vi "KeithsPhidgetAntennaOrientationFinal.vi"() -> ()   [LabVIEW 2016]
panel:
  out "Reference Elevation":sgl
  out "Reference Azimuth":dbl format="%#_13g"
  in  "Accept":bool
  in  "Don't Accept":bool
  out "Azimuth":dbl format="%#_13g"
  out "Measurements":dbl[][](array[numeric])
  in  "Antenna Power 2":dbl
  in  "Measure 2":bool
  in  "END":bool
  out "Event? 2":bool
  out "Elevation":dbl format="%#_13g"
  out "error out 2":errorcluster
  out "Attached? 2":bool
  out "Serial Number 2":i32
  in  "Antenna Power":dbl
  in  "Home":bool
  in  "Measure":bool
  out "error out":errorcluster
  out "Event?":bool
  out "Attached?":bool
  out "Serial Number":i32
  # "Reference Azimuth and Elevation"
  # "Azimuth, Elevation and Power"
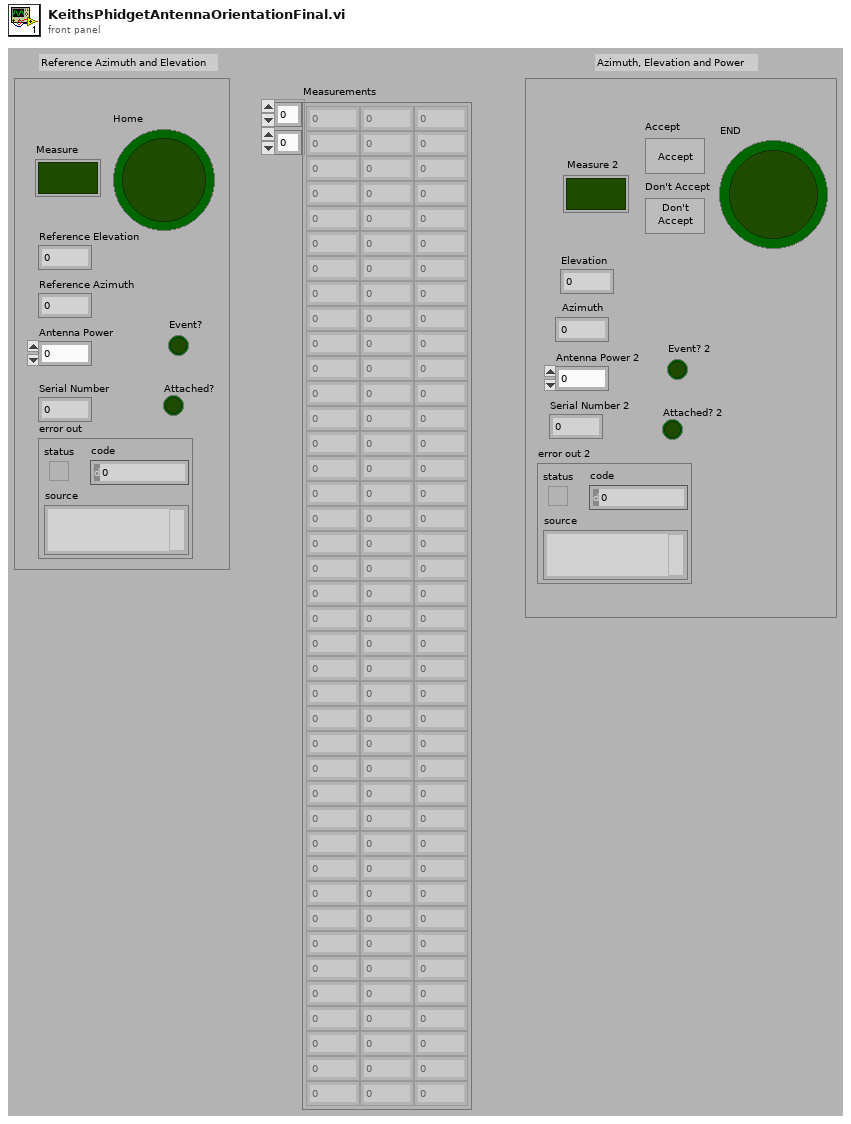
[diagram p1: front panel]
types:
  T1 = cluster{"acc0":dbl, "acc1":dbl, "acc3":dbl, "ang0":dbl, "ang1":dbl, "ang2":dbl, "mag0":dbl, "mag1":dbl, "mag2":dbl, "sec":i32, "micsec":i32}
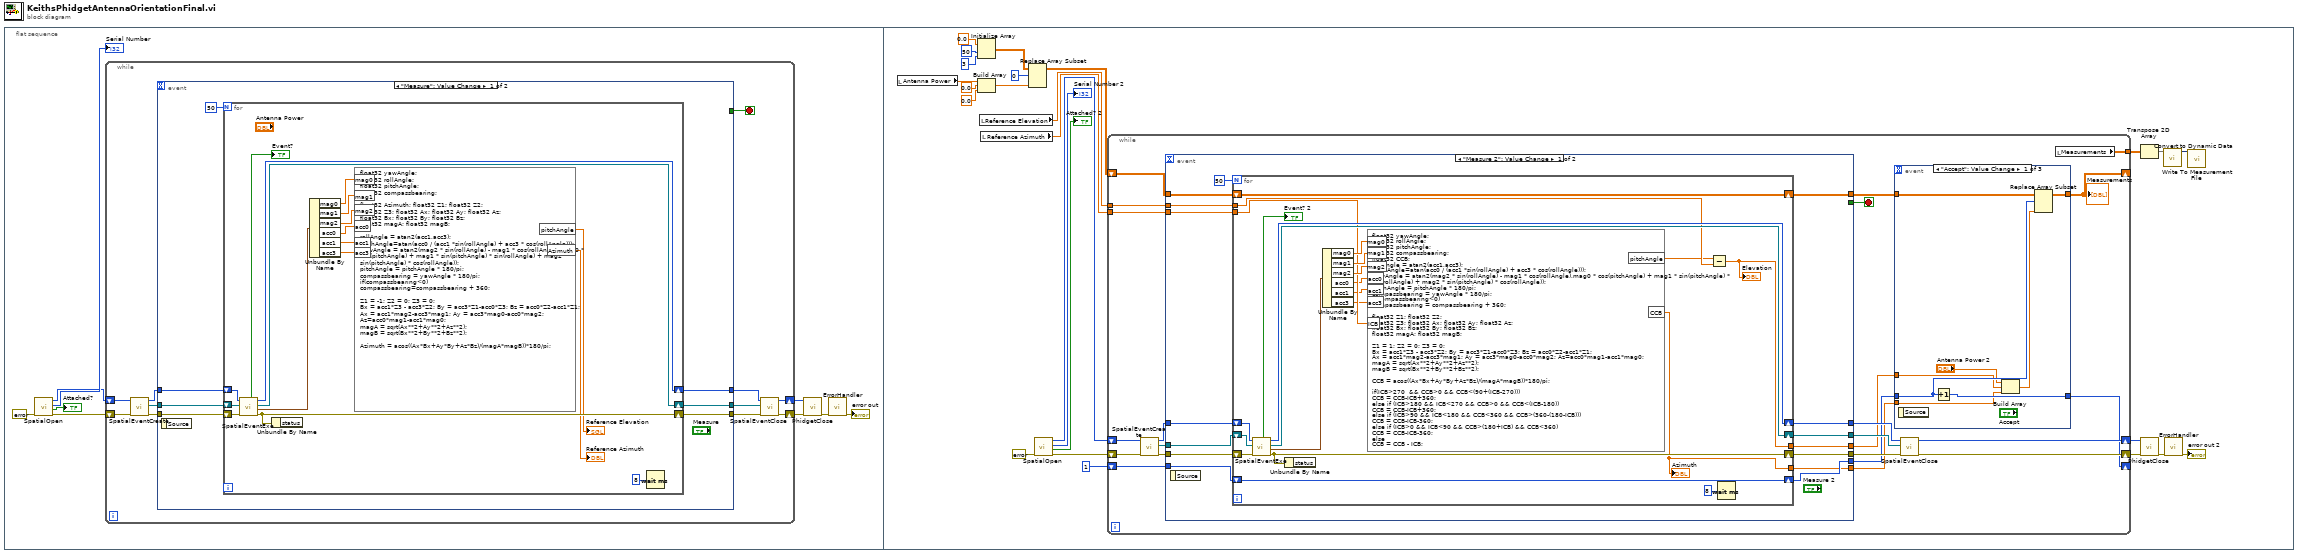
[diagram p0: block diagram]
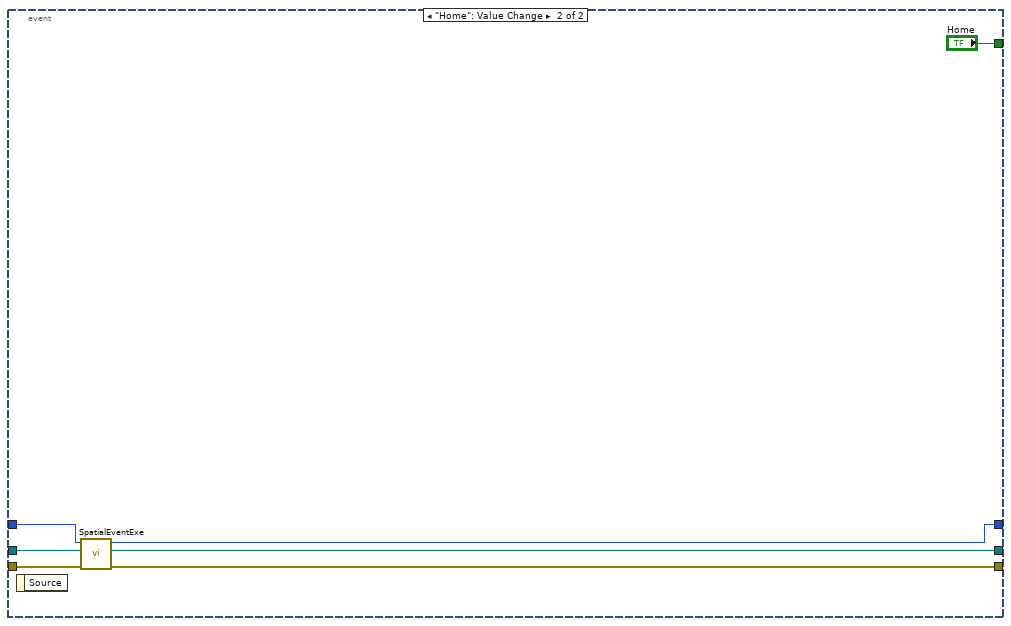
[diagram p2: hidden frame]
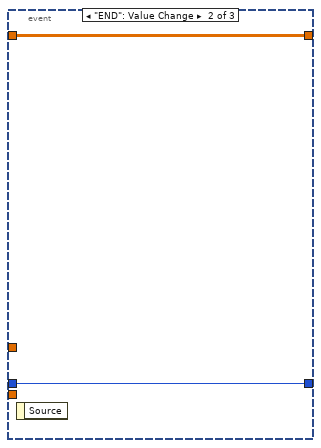
[diagram p3: hidden frame]
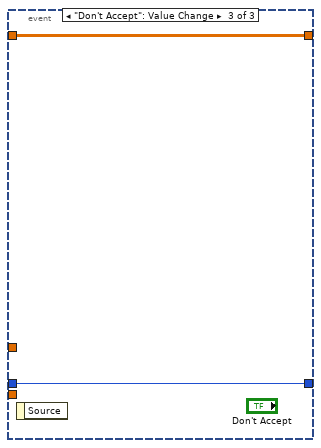
[diagram p4: hidden frame]
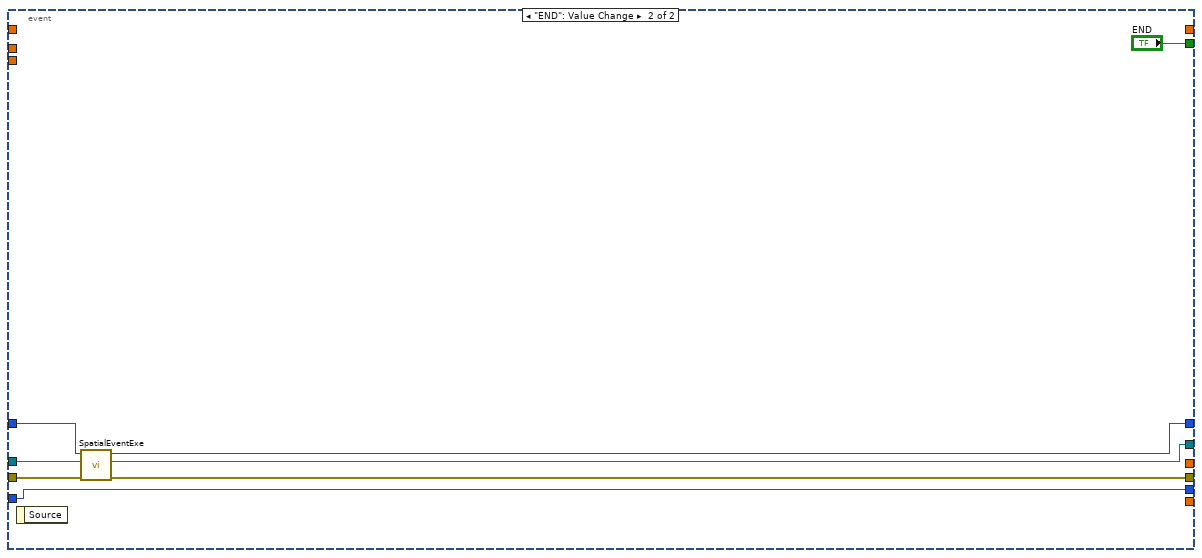
[diagram p5: hidden frame]
diagram:
  n1 = flat-sequence {
    frame #0 {
      n2 = call "SpatialOpen.vi"("error in (no error)"=errorcluster {"status"=FALSE, "code"=0, "source"=""}) -> ("error out"=w3:errorcluster, "Attached?"=→"Attached?":bool, "Serial Number Return"=→"Serial Number":i32, "Device Out"=w4:i64)  [unwired: 7 in]
      n3 = while {
        shift-right: [w18] -> w2
        shift-left: w4 -> [w20]
        shift-right: [w17] -> w1
        shift-left: w3 -> [w19]
        stop <- w10 stop-if-true
        n4 = call "SpatialEventCreate.vi"("error in (no error)"=w19, "Device In"=w20) -> ("error out"=w11:errorcluster, "Event Registration Refnum Out"=w12:refnum<event-registration>, "Device Out"=w13:i64)  [unwired: 7 in]
        n5 = event shown="[0] \"Measure\": Value Change" {
          selector: _ -> [_ _]
          dyn-events: _ -> [_ _]
          timeout: _ -> [_ _]
          tunnel: [w26 w46] -> w14
          tunnel: [w27 w45] -> w16
          tunnel: [w25 w47] -> w15
          tunnel: w13 -> [w23 w50]
          tunnel: w12 -> [w22 w49]
          tunnel: w11 -> [w21 w48]
          tunnel: [_ "Home"] -> w10
          event "Measure": Value Change {
            n6 = event-data() -> ()  [unwired: 1 in, 1 out]
            n7 = for {
              N: 50 -> [_]
              shift-right: [w37] -> w27
              shift-left: w23 -> [w42]
              shift-right: [w38] -> w26
              shift-left: w22 -> [w41]
              shift-right: [w39] -> w25
              shift-left: w21 -> [w40]
              n8 = call "SpatialEventExe.vi"("error in (no error)"=w40, "Event Registration Refnum In"=w41, "Device In"=w42) -> ("error out"=w39:errorcluster, "Output"=w36:T1, "Event Registration Refnum Out"=w38:refnum<event-registration>, "Device Out"=w37:i64, "Event?"=→"Event?":bool)  [unwired: 4 in]
              n9 = Unbundle By Name(w39) -> ()  [unwired: 1 out]
              n10 = Unbundle By Name(w36) -> ("mag0"=w35:dbl, "mag1"=w34:dbl, "mag2"=w33:dbl, "acc0"=w29:dbl, "acc1"=w30:dbl, "acc3"=w31:dbl)
              n11 = formula code="float32 yawAngle;\nfloat32 rollAngle;\nfloat32 pitchAngle;\nfloat32 compassbearing;\n\nfloat32 Azimuth; float32 Z1; float32 Z2;\nfloat32 Z3; float32 Ax; float32 Ay; float32 Az; \nfloat32 Bx; float32 By; float32 Bz;\nfloat32 magA; float32 magB;\n\nrollAngle = atan2(acc1,acc3);\npitchAngle=atan(acc0 / (acc1 *sin(rollAngle) + acc3 * cos(rollAngle)));\nyawAngle = atan2(mag2 * sin(rollAngle) - mag1 * cos(rollAngle),mag0 * cos(pitchAngle) + mag1 * sin(pitchAngle) * sin(rollAngle) + mag2 * sin(pitchAngle) * cos(rollAngle));\npitchAngle = pitchAngle * 180/pi;\ncompassbearing = yawAngle * 180/pi;\nif(compassbearing<0)\ncompassbearing=compassbearing + 360;\n\nZ1 = -1; Z2 = 0; Z3 = 0;\nBx = acc1*Z3 - acc3*Z2; By = acc3*Z1-acc0*Z3; Bz = acc0*Z2-acc1*Z1;\nAx = acc1*mag2-acc3*mag1; Ay = acc3*mag0-acc0*mag2; Az=acc0*mag1-acc1*mag0;\nmagA = sqrt(Ax**2+Ay**2+Az**2);\nmagB = sqrt(Bx**2+By**2+Bz**2);\n\nAzimuth = acos((Ax*Bx+Ay*By+Az*Bz)/(magA*magB))*180/pi;"("mag0"=w35, "mag1"=w34, "mag2"=w33, "acc0"=w29, "acc1"=w30, "acc3"=w31) -> ("Azimuth"=→"Reference Azimuth":sgl, "pitchAngle"=→"Reference Elevation":sgl)
              n12 = Wait (ms)(milliseconds to wait=u32 8) -> ()  [unwired: 1 out]
            }
          }
          event "Home": Value Change {
            n13 = event-data() -> ()  [unwired: 1 in, 1 out]
            n14 = call "SpatialEventExe.vi"("error in (no error)"=w48, "Event Registration Refnum In"=w49, "Device In"=w50) -> ("error out"=w47:errorcluster, "Event Registration Refnum Out"=w46:refnum<event-registration>, "Device Out"=w45:i64)  [unwired: 4 in, 2 out]
          }
        }
        n15 = call "SpatialEventClose.vi"("error in (no error)"=w15, "Event Registration Refnum In"=w14, "Device In"=w16) -> ("error out"=w17:errorcluster, "Device Out"=w18:i64)  [unwired: 7 in]
      }
      n16 = call "PhidgetClose.vi"("error in"=w1, "Device In"=w2) -> ("error out"=w6:errorcluster)  [unwired: 9 in]
      n17 = call "ErrorHandler.vi"("error in"=w6) -> ("error out"=→"error out":errorcluster)  [unwired: 9 in, 1 out]
    }
    frame #1 {
      n18 = local read "Antenna Power"() -> (w63:dbl)
      n19 = Initialize Array(0.0 ("element"), 50 ("dimension size"), 3 ("dimension size")) -> (w59:dbl[][])
      n20 = Build Array(w63, 0.0 ("element"), 0.0 ("element")) -> (w56:dbl[])
      n21 = local read "Reference Elevation"() -> (w52:sgl)
      n22 = local read "Reference Azimuth"() -> (w64:dbl)
      n23 = Replace Array Subset(array=w59, new element=w56, index (row)=0) -> (w58:dbl[][])  [unwired: 1 in]
      n24 = call "SpatialOpen.vi"("error in (no error)"=errorcluster {"status"=FALSE, "code"=0, "source"=""}) -> ("error out"=w71:errorcluster, "Attached?"=→"Attached? 2":bool, "Serial Number Return"=→"Serial Number 2":i32, "Device Out"=w70:i64)  [unwired: 7 in]
      n25 = while {
        shift-right: [w96] -> w69
        shift-left: w70 -> [w98]
        shift-right: [w95] -> w68
        shift-left: w71 -> [w97]
        shift-right: [w83] -> _
        shift-left: 1 -> [w87]
        shift-right: [w79] -> _
        shift-left: w58 -> [w88]
        tunnel: w64 -> [w86]
        tunnel: [w77] -> w53
        tunnel: w52 -> [w78]
        stop <- w80 stop-if-true
        n26 = call "SpatialEventCreate.vi"("error in (no error)"=w97, "Device In"=w98) -> ("error out"=w89:errorcluster, "Event Registration Refnum Out"=w90:refnum<event-registration>, "Device Out"=w91:i64)  [unwired: 7 in]
        n27 = event shown="[0] \"Measure 2\": Value Change" {
          selector: _ -> [_ _]
          dyn-events: _ -> [_ _]
          timeout: _ -> [_ _]
          tunnel: [w125 w151] -> w94
          tunnel: [w124 w149] -> w93
          tunnel: [w123 w150] -> w92
          tunnel: w91 -> [w121 w154]
          tunnel: w90 -> [w120 w153]
          tunnel: w89 -> [w119 w152]
          tunnel: w88 -> [w117 _]
          tunnel: w87 -> [w118 w148]
          tunnel: w86 -> [w116 _]
          tunnel: [_ "END"] -> w80
          tunnel: [w115 w148] -> w85
          tunnel: [w114 _] -> w84
          tunnel: [w113 _] -> w82
          tunnel: [w112 _] -> w81
          tunnel: w78 -> [w111 _]
          event "Measure 2": Value Change {
            n28 = event-data() -> ()  [unwired: 1 in, 1 out]
            n29 = for {
              N: 50 -> [_]
              shift-right: [w144] -> w125
              shift-left: w121 -> [w147]
              shift-right: [w142] -> w124
              shift-left: w119 -> [w145]
              shift-right: [w143] -> w123
              shift-left: w120 -> [w146]
              shift-right: [w139] -> w115
              shift-left: w118 -> [w139]
              shift-right: [w138] -> w114
              shift-left: w117 -> [w138]
              tunnel: w116 -> [w133]
              tunnel: [w126] -> w113
              tunnel: [w132] -> w112
              tunnel: w111 -> [w128]
              n30 = call "SpatialEventExe.vi"("error in (no error)"=w145, "Event Registration Refnum In"=w146, "Device In"=w147) -> ("error out"=w142:errorcluster, "Output"=w137:T1, "Event Registration Refnum Out"=w143:refnum<event-registration>, "Device Out"=w144:i64, "Event?"=→"Event? 2":bool)  [unwired: 4 in]
              n31 = Unbundle By Name(w142) -> ()  [unwired: 1 out]
              n32 = Unbundle By Name(w137) -> ("mag0"=w136:dbl, "mag1"=w135:dbl, "mag2"=w134:dbl, "acc0"=w131:dbl, "acc1"=w130:dbl, "acc3"=w129:dbl)
              n33 = formula code="float32 yawAngle;\nfloat32 rollAngle;\nfloat32 pitchAngle;\nfloat32 compassbearing;\nfloat32 CCB;\nrollAngle = atan2(acc1,acc3);\npitchAngle=atan(acc0 / (acc1 *sin(rollAngle) + acc3 * cos(rollAngle)));\nyawAngle = atan2(mag2 * sin(rollAngle) - mag1 * cos(rollAngle),mag0 * cos(pitchAngle) + mag1 * sin(pitchAngle) * sin(rollAngle) + mag2 * sin(pitchAngle) * cos(rollAngle));\npitchAngle = pitchAngle * 180/pi;\ncompassbearing = yawAngle * 180/pi;\nif(compassbearing<0)\ncompassbearing = compassbearing + 360;\n\nfloat32 Z1; float32 Z2;\nfloat32 Z3; float32 Ax; float32 Ay; float32 Az; \nfloat32 Bx; float32 By; float32 Bz;\nfloat32 magA; float32 magB;\n\nZ1 = 1; Z2 = 0; Z3 = 0;\nBx = acc1*Z3 - acc3*Z2; By = acc3*Z1-acc0*Z3; Bz = acc0*Z2-acc1*Z1;\nAx = acc1*mag2-acc3*mag1; Ay = acc3*mag0-acc0*mag2; Az=acc0*mag1-acc1*mag0;\nmagA = sqrt(Ax**2+Ay**2+Az**2);\nmagB = sqrt(Bx**2+By**2+Bz**2);\n\nCCB = acos((Ax*Bx+Ay*By+Az*Bz)/(magA*magB))*180/pi;\n\nif(ICB>270  && CCB>0 && CCB<(90+(ICB-270)))\nCCB = CCB-ICB+360;\nelse if (ICB>180 && ICB<270 && CCB>0 && CCB<(ICB-180))\nCCB = CCB-ICB+360;\nelse if (ICB>90 && ICB<180 && CCB<360 && CCB>(360-(180-ICB)))\nCCB = CCB-ICB-360;\nelse if (ICB>0 && ICB<90 && CCB>(180+ICB) && CCB<360)\nCCB = CCB-ICB-360;\nelse\nCCB = CCB - ICB;"("acc0"=w131, "acc1"=w130, "acc3"=w129, "mag0"=w136, "mag1"=w135, "mag2"=w134, "ICB"=w133) -> ("CCB"=w132:sgl, "pitchAngle"=w127:sgl)
              "Azimuth" <- w132
              n34 = Subtract(x=w127, y=w128) -> (x-y=w126:sgl)
              "Elevation" <- w126
              n35 = Wait (ms)(milliseconds to wait=u32 8) -> ()  [unwired: 1 out]
            }
          }
          event "END": Value Change {
            n36 = event-data() -> ()  [unwired: 1 in, 1 out]
            n37 = call "SpatialEventExe.vi"("error in (no error)"=w152, "Event Registration Refnum In"=w153, "Device In"=w154) -> ("error out"=w149:errorcluster, "Event Registration Refnum Out"=w150:refnum<event-registration>, "Device Out"=w151:i64)  [unwired: 4 in, 2 out]
          }
        }
        n38 = event shown="[0] \"Accept\": Value Change" {
          selector: _ -> [_ _ _]
          dyn-events: _ -> [_ _ _]
          timeout: _ -> [_ _ _]
          tunnel: w84 -> [w106 w108 w110]
          tunnel: [w105 w108 w110] -> w79
          tunnel: w85 -> [w104 w107 w109]
          tunnel: [w103 w107 w109] -> w83
          tunnel: w82 -> [w102 _ _]
          tunnel: w81 -> [w101 _ _]
          event "Accept": Value Change {
            n39 = event-data() -> ()  [unwired: 1 in, 1 out]
            n40 = Increment(x=w104) -> (x+1=w103:i32)
            n41 = Build Array("Antenna Power 2", w102, w101) -> (w100:dbl[])
            n42 = Replace Array Subset(array=w106, new element=w100, index (row)=w104) -> (w105:dbl[][])  [unwired: 1 in]
          }
          event "END": Value Change {
            n43 = event-data() -> ()  [unwired: 1 in, 1 out]
          }
          event "Don't Accept": Value Change {
            n44 = event-data() -> ()  [unwired: 1 in, 1 out]
          }
        }
        "Measurements" <- w79
        n45 = call "SpatialEventClose.vi"("error in (no error)"=w93, "Event Registration Refnum In"=w92, "Device In"=w94) -> ("error out"=w95:errorcluster, "Device Out"=w96:i64)  [unwired: 7 in]
        n46 = local read "Measurements"() -> (w77:dbl[][])
      }
      n47 = Transpose 2D Array(2D array=w53) -> (transposed array=w54:dbl[][])
      n48 = call "PhidgetClose.vi"("error in"=w68, "Device In"=w69) -> ("error out"=w73:errorcluster)  [unwired: 9 in]
      n49 = call "Convert to Dynamic Data"("2D Array"=w54) -> ("Dynamic Data Type"=w55:dynamicdata)  [unwired: 3 in]
      n50 = call "ErrorHandler.vi"("error in"=w73) -> ("error out"=→"error out 2":errorcluster)  [unwired: 9 in, 1 out]
      n51 = call "Write To Measurement File"("Signals"=w55) -> ()  [unwired: 16 in, 3 out]
    }
  }
